vi "Write dc.vi"(8 "error in (no error)":errorcluster, 10 "dc":dbl, 11 "Update Blue DC in":refnum<class "Update Blue DC.lvclass">) -> (0 "error out":errorcluster, 3 "Update Blue DC out":refnum<class "Update Blue DC.lvclass">)   [LabVIEW 2014, in "eCRDS Library.lvlib" / "Update Blue DC.lvclass"]
uses:
  Update Blue DC.lvclass
  Update Blue DC.lvclass/Update Blue DC.ctl
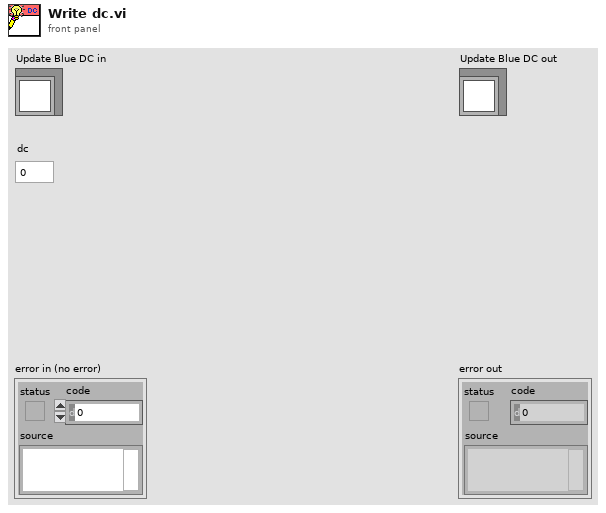
[diagram p1: front panel]
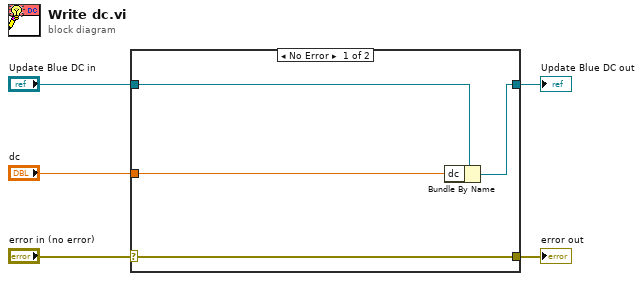
[diagram p0: block diagram]
diagram:
  n1 = case shown="No Error" "error in (no error)" {
    selector: "error in (no error)" -> [w9 w10]
    tunnel: [w9 w10] -> w4
    tunnel: [w7 w11] -> w2
    tunnel: "Update Blue DC in" -> [w8 w11]
    tunnel: "dc" -> [w6 _]
    frame No Error {
      n2 = Bundle By Name(cluster=w8, "dc"=w6) -> (w7:refnum<class "Update Blue DC.lvclass">)
    }
    frame Error {
    }
  }
  "error out" <- w4
  "Update Blue DC out" <- w2
